vi "shader_source_packet.vi"(10 ">50 Spots":bool) -> (3 "Shader Source,":string)   [LabVIEW 2019]
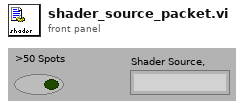
[diagram p1: front panel]
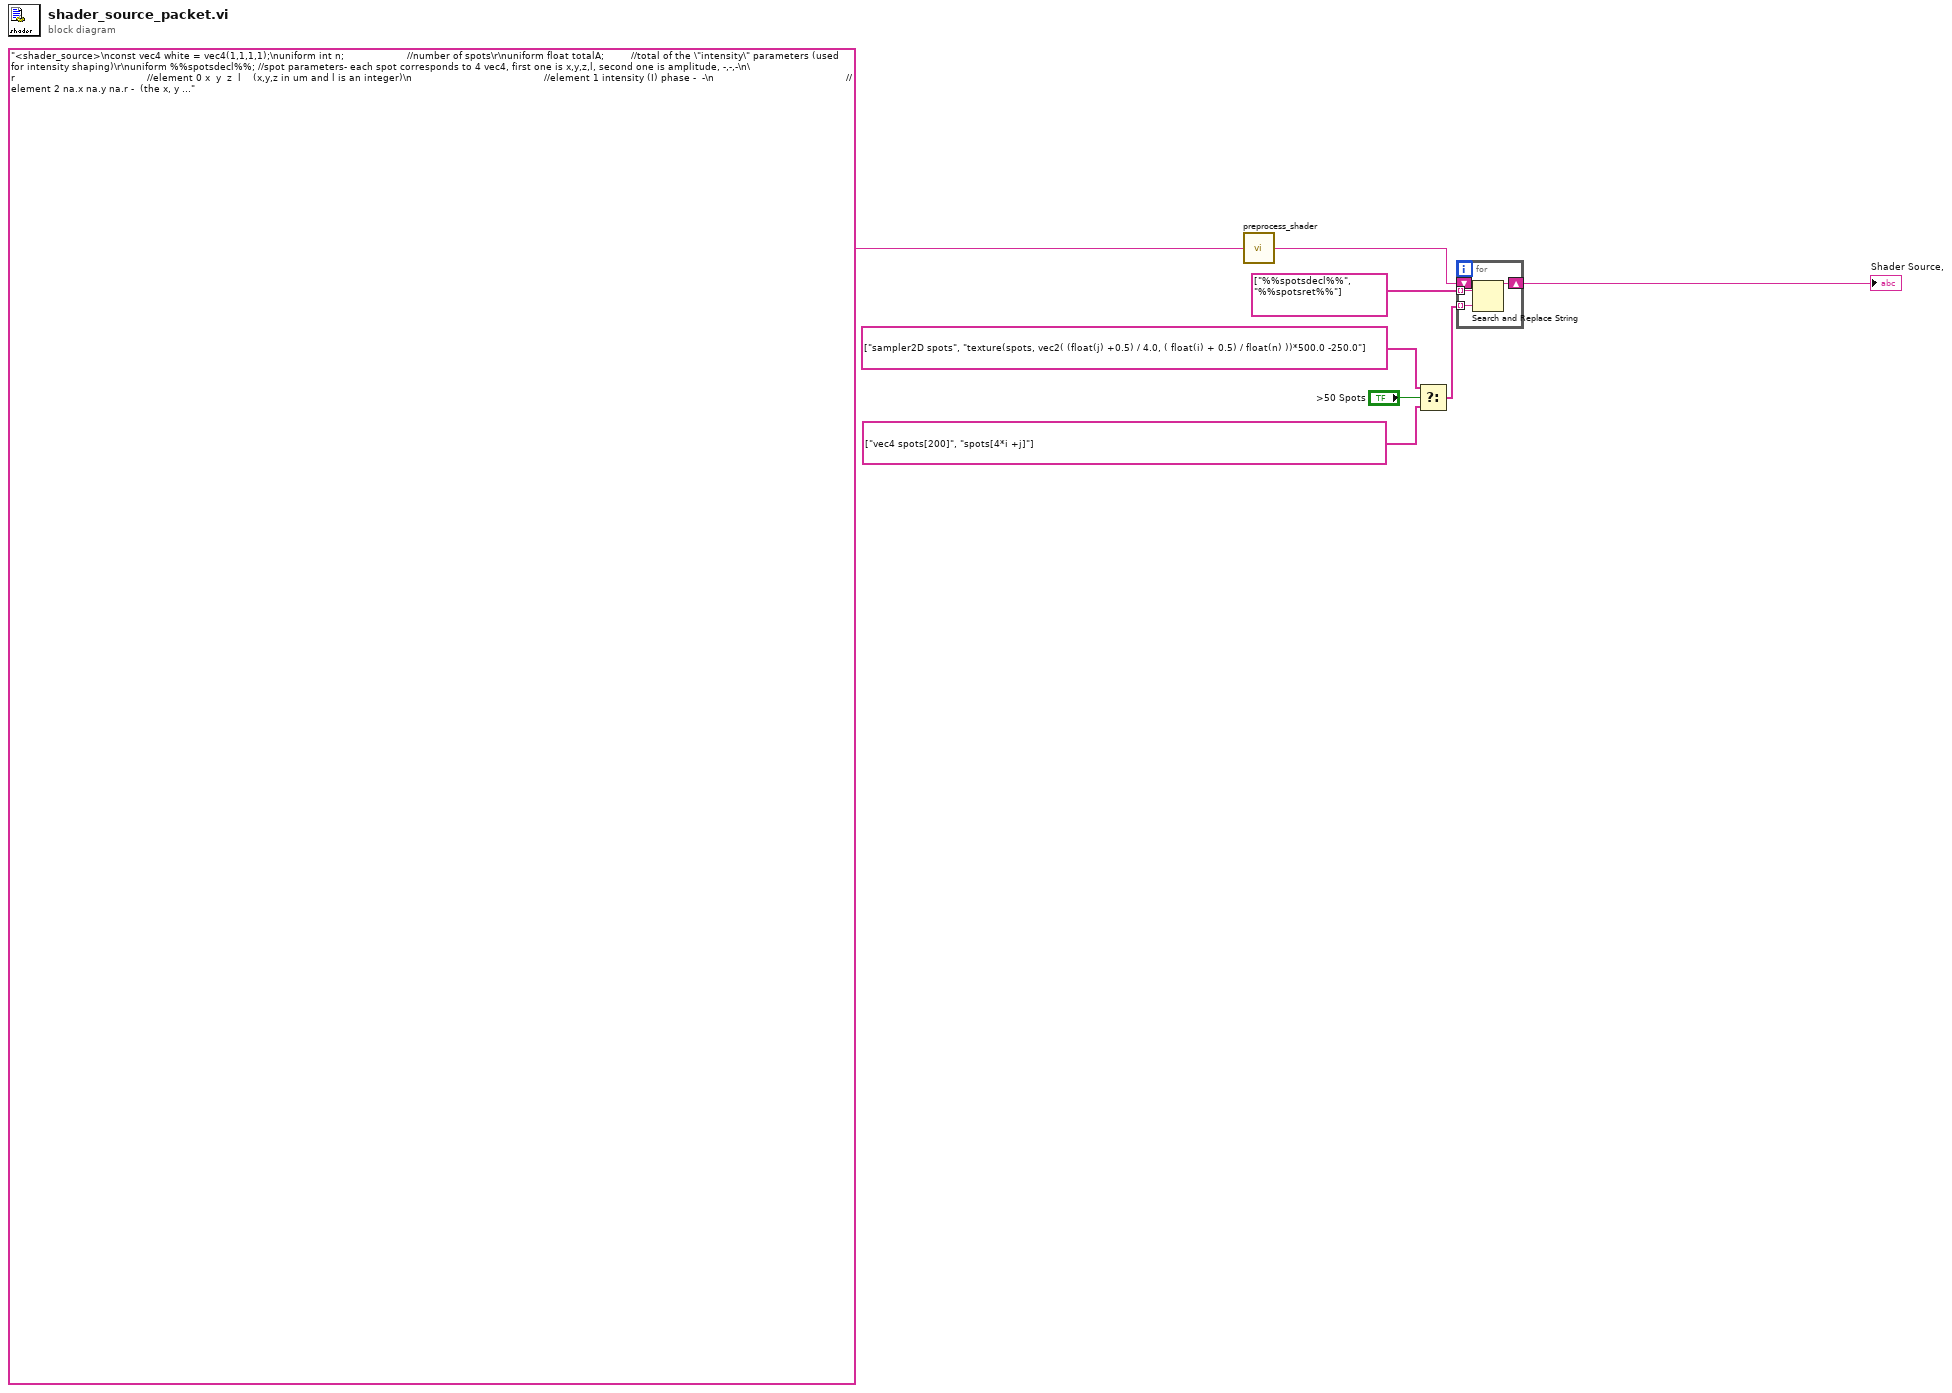
[diagram p0: block diagram]
diagram:
  n1 = call "preprocess_shader.vi"("Shader In"="<shader_source>\nconst vec4 white = vec4(1,1,1,1);\nuniform int n;                     //number of spots\r\nuniform float totalA;         //total of the \"intensity\" parameters (used for intensity shaping)\r\nuniform %%spotsdecl%%; //spot parameters- each spot corresponds to 4 vec4, first one is x,y,z,l, second one is amplitude, -,-,-\n\r                                            //element 0 x  y  z  l    (x,y,z in um and l is an integer)\n                                            //element 1 intensity (I) phase -  -\n                                            //element 2 na.x na.y na.r -  (the x, y position, and radius, of the spot on the SLM- useful for Shack-Hartmann holograms)\n                                            //element 3 line trapping x y z and phase gradient.  xyz define the size and angle of the line, phase gradient (between +/-1) is the\n                                            //scattering force component along the line.  Zero is usually a good choice for in-plane line traps\nuniform vec2 centre;        //=vec2(0.5,0.5);//centre of the hologram as a fraction of its size (usually 0.5,0.5)\r\nuniform vec2 size;            //=vec2(7000,7000);//size of the hologram in microns\r\nuniform float f;                 //=1600; //focal length in microns\r\nuniform float k;                //=9.36; //wavevector in 1/microns\r\nuniform float blazing[32]; //blazing function\r\nuniform float zernikeCoefficients[12]; //zernike coefficients, matching the modes defined below\nuniform vec3 zernx;        //=vec3(0.0,0.0,0.0);\nuniform vec3 zerny;        //=vec3(0.0,0.0,0.0);\nuniform vec3 zernz;        //=vec3(0.0,0.0,0.0);\r\n%%standardfunctions%%\n\nvec4 spot(int i, int j){\n  return %%spotsret%%;\n}\n\nvoid main(void)\r\n{\r\n   float phase;                                                       //phase of current pixel, due to the spot (in loop) or of the resultant hologram (after loop)\r\n   float amplitude;                                               //ditto for amplitude\r\n   vec2 xy=(gl_TexCoord[0].xy-centre)*size;    //current xy position in the hologram, in microns\r\n   float phi=atan(xy.x,xy.y);\t\t                              //angle of the line joining our point to the centre of the pattern\r\n   float length;                                                     //length of a line\r\n   vec4 pos=vec4(xy/f,1.0-dot(xy,xy)/2.0/f/f,phi/k);\r\n   vec4 na;                                                           //to be used later, inside the loop\r\n\t float sx;\r\n\n                                                     //this loop goes through the spots and calculates the contribution from each one, summing\n                                                                            //real and imaginary parts as we go.\n\r   vec2 total = vec2(0.0,0.0);                             //real and imaginary parts of the complex hologram for this pixel\n   for(int i=0; i<n; i++){\n      amplitude=spot(i,1)[0];                             //amplitude of current spot\r\n      phase=k*dot(spot(i,0),pos)+spot(i,1)[1]; \n                                                                            //this is the basic gratings and lenses algorithm; phase=kx*x+ky*y+kz*(x^2+y^2)+l*theta\n\n      na = spot(i,2);                                           //restrict the spot to a region of the back aperture which is na[2] in radius, centred on na.xy\r\n      if(dot(na.xy-xy/size,na.xy-xy/size) > na[2]*na[2]){\n        amplitude = 0.0;\n      }\n//creates an xyz line trap, needs amplitude shaping.\n\r      vec4 line = spot(i,3);\n      length=sqrt(dot(line.xyz,line.xyz));\r\n      if(length>0.0){\r\n\t\t      sx=k*dot(vec4(pos.xyz,1.0*length),line);\r\n\t\t      if(sx!=0.0) amplitude*=sin(sx)/sx;\r\n      }\n\n      total += amplitude * unitvector(phase); //finally, convert from amplitude+phase to real+imaginary for the summation\r\n   }\n   amplitude = dot(total, total);\r\n   phase=atan(total.y,total.x);\r\n   phase += zernikeAberration(); //apply aberration correction\n   if(amplitude==0.0) phase=0.0;                                      //don't focus zero order\r\n   if(totalA>0.0){ //do amplitude-shaping (dumps light into zero order when not needed)\r\n     phase *= clamp(amplitude/totalA,0.0,1.0);\r\n   }\r\n   phase = wrap2pi(phase);\r\n//   gl_FragColor = gray_to_16bit( apply_LUT(phase)); //16-bit output with LUT\n   gl_FragColor = vec4(1,1,1,1) * apply_LUT(phase);  //8-bit output with LUT\n//   gl_FragColor = vec4(1,1,1,1) * phase_to_gray(phase);          //8-bit output, linear LUT\n//   gl_FragColor = clamp(vec4(.866*cos(phase) -.5*sin(phase), -.866*cos(phase)-.5*sin(phase),sin(phase),1.0)/1.5+0.6667,0.0,1.0); //phase rainbow output\n//   gl_FragColor = vec4(%%randcol%%);\n\n}\n</shader_source>\n\n<swap_buffers_at_refresh_rate>\n0\n</swap_buffers_at_refresh_rate>\n<network_reply>\n1\n</network_reply>\n</data>") -> ("Shader Out"=w7:string)
  n2 = Select(t=string[] ["sampler2D spots", "texture(spots, vec2( (float(j) +0.5) / 4.0, ( float(i) + 0.5) / float(n) ))*500.0 -250.0"], s=">50 Spots", f=string[] ["vec4 spots[200]", "spots[4*i +j]"]) -> (s? t:f=w3:string[])
  n3 = for {
    tunnel: string[] ["%%spotsdecl%%", "%%spotsret%%"] -> [w12] mode=indexing
    tunnel: w3 -> [w11] mode=indexing
    shift-right: [w9] -> w6
    shift-left: w7 -> [w10]
    n4 = Search and Replace String(input string=w10, search string=w12, replace string=w11) -> (result string=w9:string)  [unwired: 5 in, 3 out]
  }
  "Shader Source," <- w6
